vi "Close.vi"(8 "error in (no error)":errorcluster, 11 "TTL in":refnum<class "TTL.lvclass">) -> (0 "error out":errorcluster, 3 "TTL out":refnum<class "TTL.lvclass">)   [LabVIEW 2011, in "TTL.lvclass"]
uses:
  TTL.lvclass
  TTL.lvclass/TTL.ctl
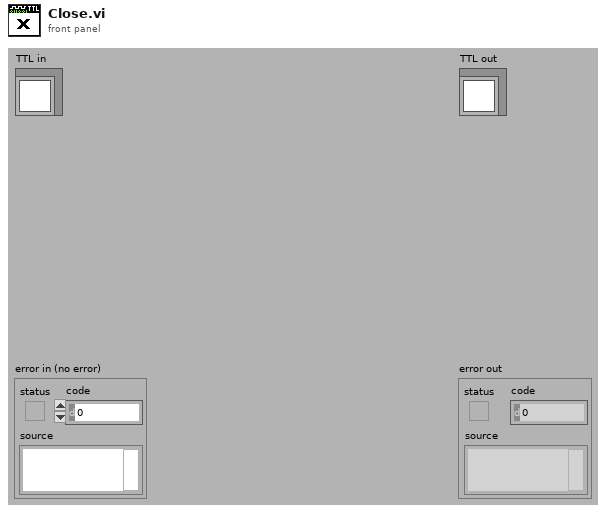
[diagram p1: front panel]
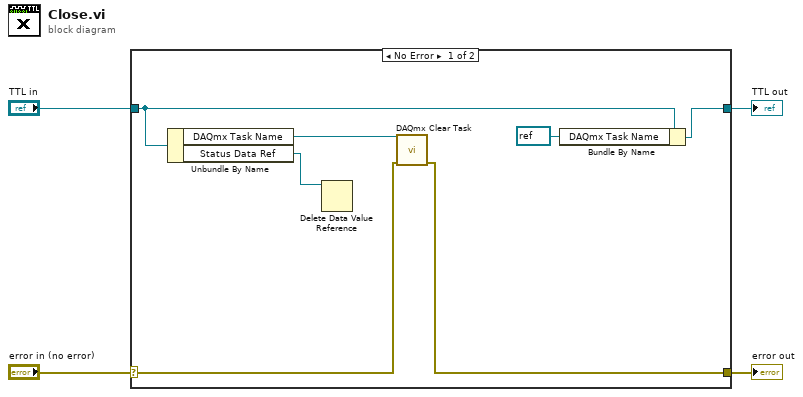
[diagram p0: block diagram]
diagram:
  n1 = case shown="No Error" "error in (no error)" {
    selector: "error in (no error)" -> [w10 w13]
    tunnel: [w9 w13] -> w3
    tunnel: [w7 w12] -> w1
    tunnel: "TTL in" -> [w8 w12]
    frame No Error {
      n2 = Unbundle By Name(w8) -> ("DAQmx Task Name"=w11:refnum<k21>, "Status Data Ref"=w5:refnum<data-value>)
      n3 = Delete Data Value Reference(data value reference=w5) -> ()  [unwired: 1 in, 2 out]
      n4 = call <vilib>:"DAQmx Clear Task.vi"("task in"=w11, "error in"=w10) -> ("error out"=w9:errorcluster)  [unwired: 13 in]
      n5 = Bundle By Name(cluster=w8, "DAQmx Task Name"=refnum<k21> refnum) -> (w7:refnum<class "TTL.lvclass">)
    }
    frame Error {
    }
  }
  "error out" <- w3
  "TTL out" <- w1
